vi "Drop.vi"(6 "Copy?":bool, 7 "BetterHandle in (source)":refnum<class "BetterHandle.lvclass">, 8 "error in (no error)":errorcluster, 9 "Coords":T1, 10 "BetterDropOp":refnum<class "BetterDropOp.lvclass">, 11 "BetterHandle in (destination)":refnum<class "BetterHandle.lvclass">) -> (0 "error out":errorcluster, 3 "BetterHandle out (destination)":refnum<class "BetterHandle.lvclass">, 5 "BetterHandle out (source)":refnum<class "BetterHandle.lvclass">)   [LabVIEW 2020, in "BetterDragAndDrop.lvlib" / "BetterHandle.lvclass"]
uses:
  BetterHandle.lvclass
  <vilib>/Utility/miscctls.llb/LVPoint32TypeDef.ctl
  BetterDropOp/BetterDropOp.lvclass
  BetterHandle.lvclass/BetterHandle.ctl
  BetterTreeBar/SubVIs/Horizontal Bar Enumeration.ctl
  BetterTreeBar/BetterHorizontalBar.lvclass
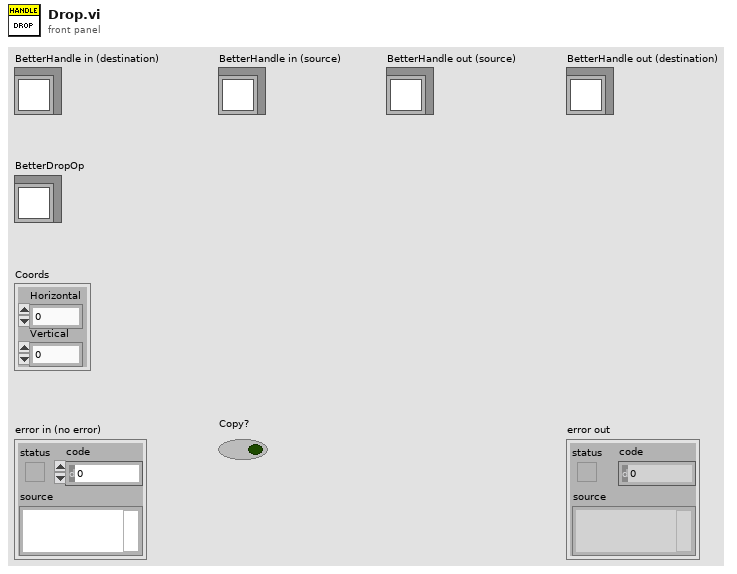
[diagram p1: front panel]
types:
  T1 = typedef "LVPoint32TypeDef.ctl" = cluster{"Horizontal":i32, "Vertical":i32}
  T2 = typedef "BetterDragAndDrop.lvlib/BetterHorizontalBar.lvclass/Horizontal Bar Enumeration.ctl" = enum16{"None", "only bar", "tilda up"}
  T3 = typedef "BetterDragAndDrop.lvlib/BetterHandle.lvclass/DragOver Output.ctl" = cluster{"Displayed Row":i32, "Position":T4, "Row's TreeItem index":i32, "indent":i32, "Accepted?":bool, "Insertion index":i32, "Top left visible TreeItem index":i32, "Bar type":T2}
  T4 = typedef "BetterDragAndDrop.lvlib/BetterHandle.lvclass/DragOverPosition.ctl" = enum16{"On Row", "Inbetween"}
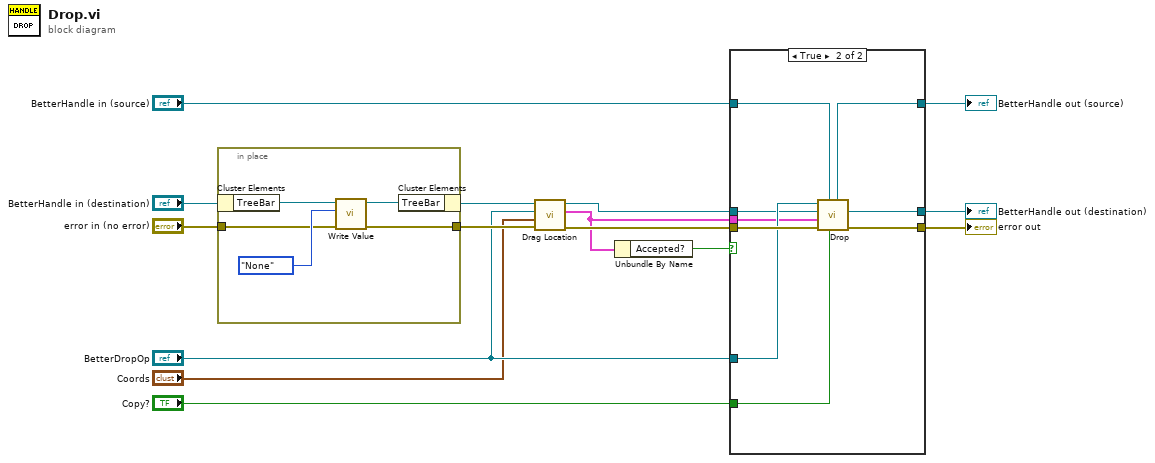
[diagram p0: block diagram]
diagram:
  n1 = in-place {
    in-place-border: "error in (no error)" -> [w17]
    in-place-border: [w16] -> w10
    n2 = in-place-cluster #1("BetterHandle in (destination)") -> ("TreeBar"=w20:refnum<class "BetterHorizontalBar.lvclass">)
    n3 = call "Write Value.vi"("error in (no error)"=w17, "New Value"=Horizontal_Bar_Enumeration."None", "BetterTreeBar in"=w20) -> ("error out"=w16:errorcluster, "BetterTreeBar out"=w18:refnum<class "BetterHorizontalBar.lvclass">)  [unwired: 7 in]
    n4 = in-place-cluster #1("TreeBar"=w18) -> (w15:refnum<class "BetterHandle.lvclass">)
  }
  n5 = call-dynamic "Drag Location.vi"("error in (no error)"=w10, "Coords"="Coords", "BetterDropOp"="BetterDropOp", "BetterHandle in"=w15) -> ("error out"=w14:errorcluster, "DragOver Output"=w12:T3, "BetterHandle out"=w13:refnum<class "BetterHandle.lvclass">)  [unwired: 5 in]
  n6 = Unbundle By Name(w12) -> ("Accepted?"=w11:bool)
  n7 = case shown="True" w11 {
    tunnel: w14 -> [w22 w32]
    tunnel: "BetterDropOp" -> [_ w31]
    tunnel: "BetterHandle in (source)" -> [w21 w30]
    tunnel: [w21 w29] -> w6
    tunnel: w13 -> [w23 w28]
    tunnel: w12 -> [_ w27]
    tunnel: "Copy?" -> [_ w26]
    tunnel: [w23 w25] -> w5
    tunnel: [w22 w24] -> w2
    frame False {
    }
    frame True {
      n8 = call-dynamic "Drop.vi"("Copy?"=w26, "BetterHandle in (source)"=w30, "error in (no error)"=w32, "DragOver Output"=w27, "BetterHandle in (destination)"=w28, "BetterDropOp in"=w31) -> ("error out"=w24:errorcluster, "BetterHandle out (destination)"=w25:refnum<class "BetterHandle.lvclass">, "BetterHandle out (source)"=w29:refnum<class "BetterHandle.lvclass">)  [unwired: 2 in, 1 out]
    }
  }
  "error out" <- w2
  "BetterHandle out (destination)" <- w5
  "BetterHandle out (source)" <- w6
